vi "Obtain Request Events.vi"(8 "error in (no error)":errorcluster, 10 "Create New?":bool) -> (0 "error out":errorcluster, 2 "Anode Request Events":T1)   [LabVIEW 2024, in "Anode.lvlib"]
doc: "This VI Obtains/Creates the Requests events that will be used for other modules to communicate with the module that owns this VI. These Requests events will be accessed only via Public API methods for this module.\n\n<b>NOTE</b>: The contents of this VI are automatically generated and modified by the <b>Tools > Delacor > DQMH</b> utilities. Consider using those utilities instead of making your own modifications to this VI.\n_____\nBased on Delacor QMH Project Template 3.1.0.34."
uses:
  Anode.lvlib
  Request Events--cluster.ctl
  Stop Argument--cluster.ctl
  Show Panel Argument--cluster.ctl
  Hide Panel Argument--cluster.ctl
  Get Module Execution Status Argument--cluster.ctl
  Show Diagram Argument--cluster.ctl
  Change Panel Argument--cluster.ctl
  <vilib>/MGI/Panel Manager/Panel/Panel/Panel.lvclass
  Set Anode Inlet Pressure SP Argument--cluster.ctl
  Initialise Pressure Regulator Interface Argument--cluster.ctl
  Modbus Config--cluster.ctl
  Start Polling Pressure Regulator Status Argument--cluster.ctl
  Stop Polling Pressure Regulator Status Argument--cluster.ctl
  Read Pressure Regulator Status Argument--cluster.ctl
  Set Pressure Regulator Control Function Argument--cluster.ctl
  Modbus Flexi-Flow API/Control Function Values--enum.ctl
  Set Anode Inlet Flow SP Argument--cluster.ctl
  Set Anode Inlet Valve State Argument--cluster.ctl
  Anode Solenoid Valve--enum.ctl
  Wake Connection Helper Loop Argument--cluster.ctl
  Set Anode Gas Supply Valve Argument--cluster.ctl
  Set Purge Valve Argument--cluster.ctl
  Set Purge Strategy Argument--cluster.ctl
  Purge Strategy--cluster.ctl
  Purge Strategy--enum.ctl
  Wake Purge Strategy Helper Loop Argument--cluster.ctl
  Update Purge Strategy Settings Argument--cluster.ctl
  Wake Purge Helper Loop Argument--cluster.ctl
  Wake Recirculation Pump Helper Loop Argument--cluster.ctl
  Sleep Recirculation Pump Helper Loop Argument--cluster.ctl
  Set Pump Speed SP Argument--cluster.ctl
  Set Pump Enable State Argument--cluster.ctl
  Set Pump Speed Control Mode Argument--cluster.ctl
  Update Purge Strategy Helper Loop Argument--cluster.ctl
  Force Purge Argument--cluster.ctl
  Reset Counter Argument--cluster.ctl
  Wake H2 Sensor Loop Argument--cluster.ctl
  Sleep H2 Sensor Loop Argument--cluster.ctl
  Start H2 Sensor Measurement Argument--cluster.ctl
  Stop H2 Sensor Measurement Argument--cluster.ctl
  Modbus Flexi-Flow API/Bronkhorst Flexi-Flow ModbusTCP API.lvlib
panel:
  # "NOTE: The contents of this VI are automatically generated and modified by the Tools > Delacor > DQMH utilities. Consider using those utilities instead of making your own modifications to this VI."
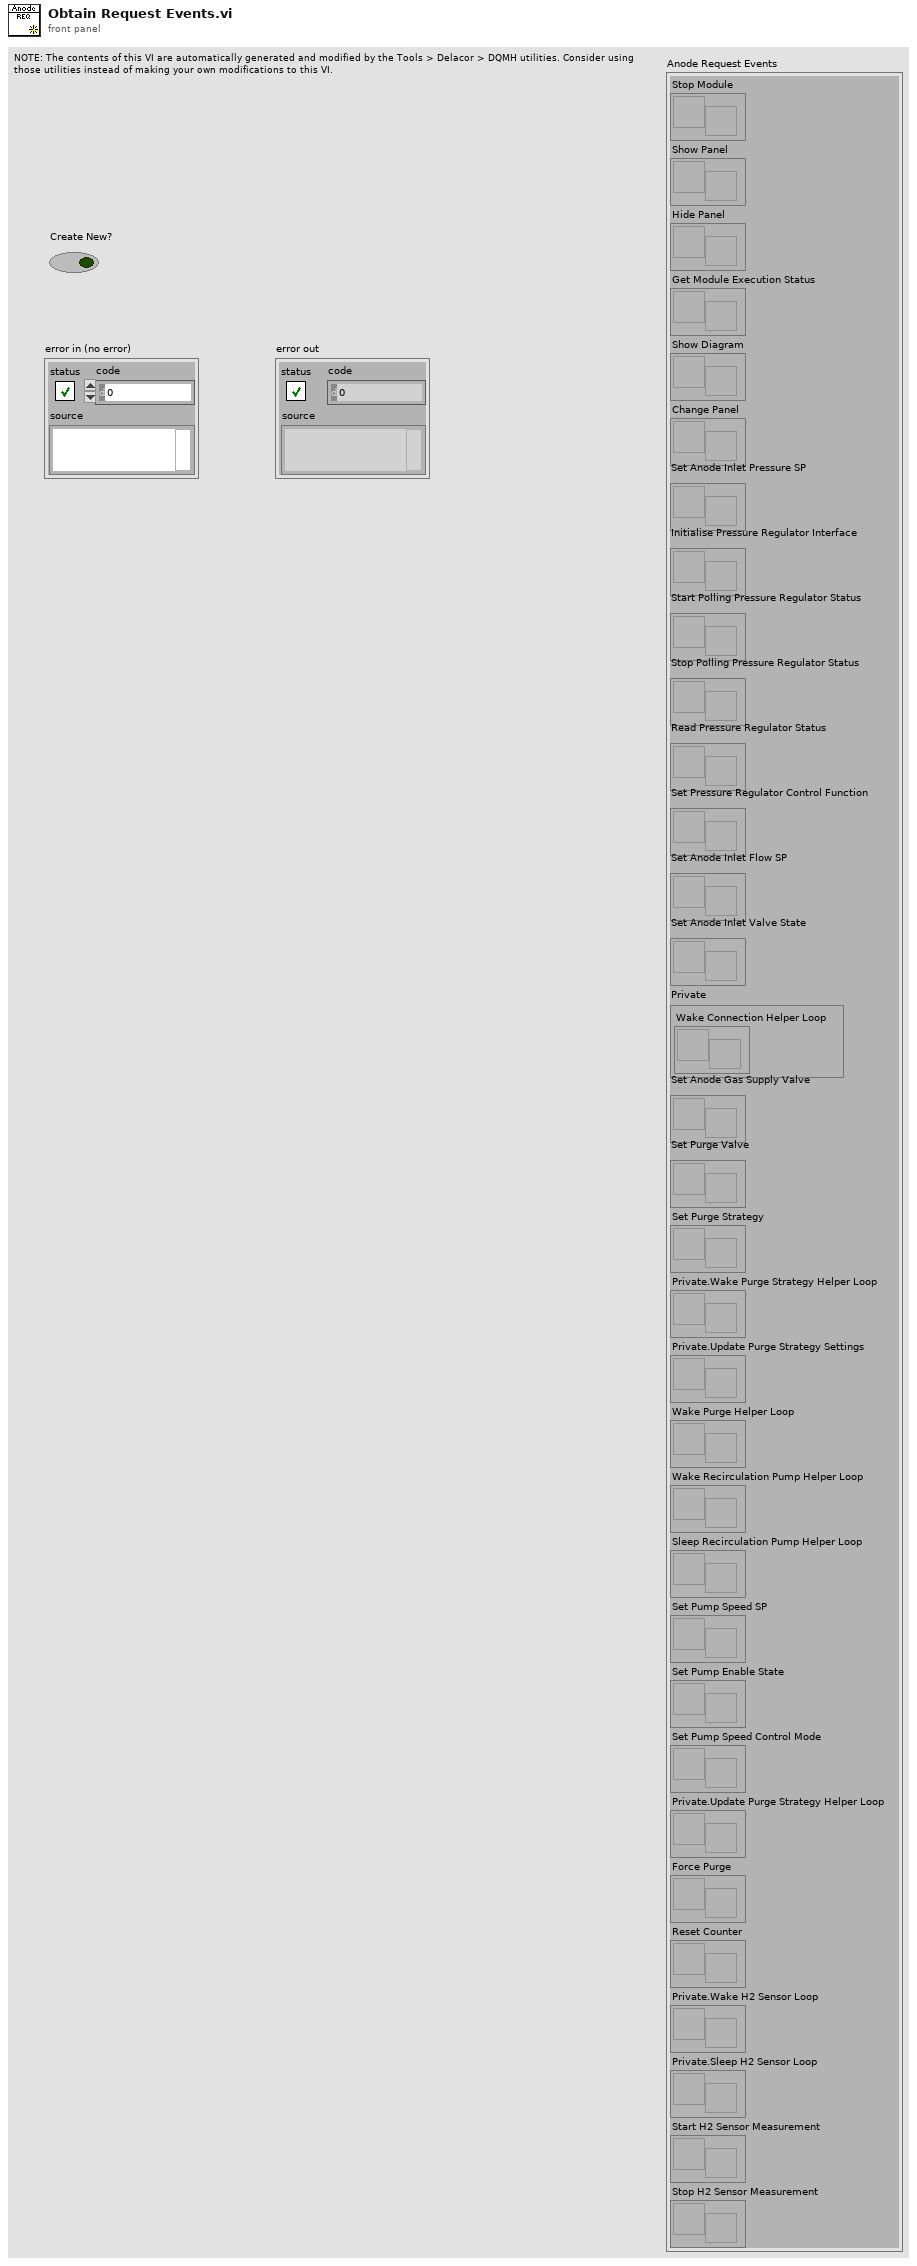
[diagram p1: front panel]
types:
  T1 = typedef "Anode.lvlib/Request Events--cluster.ctl" = cluster{"Stop Module":refnum<user-event>, "Show Panel":refnum<user-event>, "Hide Panel":refnum<user-event>, "Get Module Execution Status":refnum<user-event>, "Show Diagram":refnum<user-event>, "Change Panel":refnum<user-event>, "Set Anode Inlet Pressure SP":refnum<user-event>, "Initialise Pressure Regulator Interface":refnum<user-event>, "Start Polling Pressure Regulator Status":refnum<user-event>, "Stop Polling Pressure Regulator Status":refnum<user-event>, "Read Pressure Regulator Status":refnum<user-event>, "Set Pressure Regulator Control Function":refnum<user-event>, "Set Anode Inlet Flow SP":refnum<user-event>, "Set Anode Inlet Valve State":refnum<user-event>, "Private":cluster{"Wake Connection Helper Loop":refnum<user-event>}, "Set Anode Gas Supply Valve":refnum<user-event>, "Set Purge Valve":refnum<user-event>, "Set Purge Strategy":refnum<user-event>, "Private.Wake Purge Strategy Helper Loop":refnum<user-event>, "Private.Update Purge Strategy Settings":refnum<user-event>, "Wake Purge Helper Loop":refnum<user-event>, "Wake Recirculation Pump Helper Loop":refnum<user-event>, "Sleep Recirculation Pump Helper Loop":refnum<user-event>, "Set Pump Speed SP":refnum<user-event>, "Set Pump Enable State":refnum<user-event>, "Set Pump Speed Control Mode":refnum<user-event>, "Private.Update Purge Strategy Helper Loop":refnum<user-event>, "Force Purge":refnum<user-event>, "Reset Counter":refnum<user-event>, "Private.Wake H2 Sensor Loop":refnum<user-event>, "Private.Sleep H2 Sensor Loop":refnum<user-event>, "Start H2 Sensor Measurement":refnum<user-event>, "Stop H2 Sensor Measurement":refnum<user-event>}
  T2 = typedef "Anode.lvlib/Stop H2 Sensor Measurement Argument--cluster.ctl" = cluster{"Boolean":bool}
  T3 = typedef "Anode.lvlib/Start H2 Sensor Measurement Argument--cluster.ctl" = cluster{"Boolean":bool}
  T4 = typedef "Anode.lvlib/Sleep H2 Sensor Loop Argument--cluster.ctl" = cluster{"Boolean":bool}
  T5 = typedef "Anode.lvlib/Wake H2 Sensor Loop Argument--cluster.ctl" = cluster{"Boolean":bool}
  T6 = typedef "Anode.lvlib/Reset Counter Argument--cluster.ctl" = cluster{"Boolean":bool}
  T7 = typedef "Anode.lvlib/Force Purge Argument--cluster.ctl" = cluster{"Boolean":bool}
  T8 = typedef "Anode.lvlib/Update Purge Strategy Helper Loop Argument--cluster.ctl" = cluster{"Purge Controller":T9}
  T9 = typedef "Anode.lvlib/Purge Strategy--cluster.ctl" = cluster{"Strategy":T10, "Purge Interval [s]":dbl, "Purge Duration [s]":dbl}
  T10 = typedef "Anode.lvlib/Purge Strategy--enum.ctl" = enum16{"FORCE OFF", "FORCE ON", "TIMED"}
  T11 = typedef "Anode.lvlib/Set Pump Speed Control Mode Argument--cluster.ctl" = cluster{"Enable Speed Control":enum8{"DISABLE", "ENABLE"}}
  T12 = typedef "Anode.lvlib/Set Pump Enable State Argument--cluster.ctl" = cluster{"Enable Pump":enum16{"DISABLE", "ENABLE"}}
  T13 = typedef "Anode.lvlib/Set Pump Speed SP Argument--cluster.ctl" = cluster{"Pump Speed SP":dbl}
  T14 = typedef "Anode.lvlib/Sleep Recirculation Pump Helper Loop Argument--cluster.ctl" = cluster{"Boolean":bool}
  T15 = typedef "Anode.lvlib/Wake Recirculation Pump Helper Loop Argument--cluster.ctl" = cluster{"Boolean":bool}
  T16 = typedef "Anode.lvlib/Wake Purge Helper Loop Argument--cluster.ctl" = cluster{"Boolean":bool}
  T17 = typedef "Anode.lvlib/Update Purge Strategy Settings Argument--cluster.ctl" = cluster{"Purge Settings":T9}
  T18 = typedef "Anode.lvlib/Wake Purge Strategy Helper Loop Argument--cluster.ctl" = cluster{"Boolean":bool}
  T19 = typedef "Anode.lvlib/Set Purge Strategy Argument--cluster.ctl" = cluster{"Purge Controller":T9}
  T20 = typedef "Anode.lvlib/Set Purge Valve Argument--cluster.ctl" = cluster{"Valve State":enum16{"CLOSED", "OPEN"}}
  T21 = typedef "Anode.lvlib/Set Anode Gas Supply Valve Argument--cluster.ctl" = cluster{"Valve State":enum16{"CLOSED", "OPEN"}}
  T22 = typedef "Anode.lvlib/Wake Connection Helper Loop Argument--cluster.ctl" = cluster{"Boolean":bool}
  T23 = typedef "Anode.lvlib/Set Anode Inlet Valve State Argument--cluster.ctl" = cluster{"Anode Solenoid Valve":T24}
  T24 = typedef "Anode.lvlib/Anode Solenoid Valve--enum.ctl" = enum16{"CLOSED", "OPEN"}
  T25 = typedef "Anode.lvlib/Set Anode Inlet Flow SP Argument--cluster.ctl" = cluster{"Flow SP [slm]":dbl}
  T26 = typedef "Anode.lvlib/Set Pressure Regulator Control Function Argument--cluster.ctl" = cluster{"Function":T27}
  T27 = typedef "Bronkhorst Flexi-Flow ModbusTCP API.lvlib/Control Function Values--enum.ctl" = enum16{"Flow", "Upstream pressure", "Downstream pressure", "Flow with upstream pressure limit", "Flow with downstream pressure limit", "Upstream pressure with flow limit", "Downstream pressure with flow limit"}
  T28 = typedef "Anode.lvlib/Read Pressure Regulator Status Argument--cluster.ctl" = cluster{"Boolean":bool}
  T29 = typedef "Anode.lvlib/Stop Polling Pressure Regulator Status Argument--cluster.ctl" = cluster{"Boolean":bool}
  T30 = typedef "Anode.lvlib/Start Polling Pressure Regulator Status Argument--cluster.ctl" = cluster{"Polling Interval [ms]":i32}
  T31 = typedef "Anode.lvlib/Initialise Pressure Regulator Interface Argument--cluster.ctl" = cluster{"Modbus Config":T32}
  T32 = typedef "Anode.lvlib/Modbus Config--cluster.ctl" = cluster{"IP Address":string, "Port (502)":u16, "Slave ID (255)":u8, "Timeout (10000)":i32}
  T33 = typedef "Anode.lvlib/Set Anode Inlet Pressure SP Argument--cluster.ctl" = cluster{"Anode Inlet Pressure [bar]":dbl}
  T34 = typedef "Anode.lvlib/Change Panel Argument--cluster.ctl" = cluster{"New Panel":refnum<class "Panel.lvclass">}
  T35 = typedef "Anode.lvlib/Hide Panel Argument--cluster.ctl" = cluster{"Hide Panel?":bool}
  T36 = typedef "Anode.lvlib/Show Panel Argument--cluster.ctl" = cluster{"Show Panel?":bool}
  T37 = typedef "Anode.lvlib/Show Diagram Argument--cluster.ctl" = cluster{"Debug?":bool}
  T38 = typedef "Anode.lvlib/Get Module Execution Status Argument--cluster.ctl" = cluster{"Running?":bool}
  T39 = typedef "Anode.lvlib/Stop Argument--cluster.ctl" = cluster{"Origin":string, "Exit via Stop Module Req?":bool, "Wait for Module to stop?":bool}
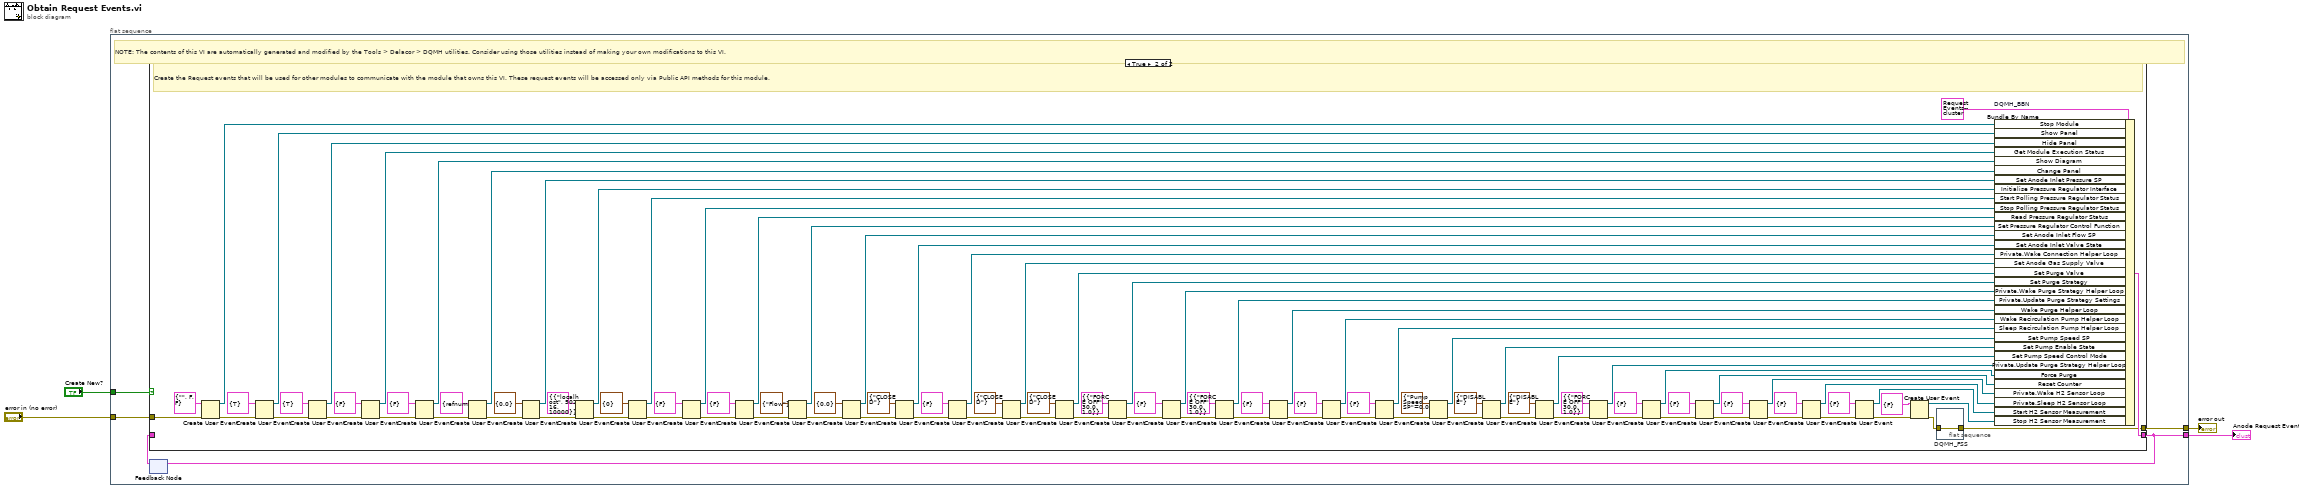
[diagram p0: block diagram]
diagram:
  n1 = flat-sequence {
    tunnel: [w9] -> w4
    tunnel: "error in (no error)" -> [w8]
    tunnel: [w6] -> w2
    tunnel: "Create New?" -> [w5]
    frame #0 {
      # "NOTE: The contents of this VI are automatically generated and modified by the Tools > Delacor > DQMH utilities. Consider using those utilities instead of making your own modifications to this VI."
      n2 = feedback #1() -> (w7:T1)  [unwired: 1 in]
      n3 = case shown="True" w5 {
        tunnel: [w10 w104] -> w9
        tunnel: w8 -> [w10 w114]
        tunnel: [w11 w111] -> w6
        tunnel: w7 -> [w11 _]
        frame False {
          # "Obtain the Request events that were created in a previous call to this VI."
        }
        frame True {
          # "Create the Request events that will be used for other modules to communicate with the module that owns this VI. These request events will be accessed only via Public API methods for this module."
          n4 = Create User Event(user event datatype=T39 {"Origin"="", "Exit via Stop Module Req?"=FALSE, "Wait for Module to stop?"=FALSE} ("Stop Argument"), error in=w114) -> (user event=w112:refnum<user-event>, error out=w109:errorcluster)
          n5 = Create User Event(user event datatype=T36 {"Show Panel?"=TRUE} ("Show Panel Argument"), error in=w109) -> (user event=w108:refnum<user-event>, error out=w107:errorcluster)
          n6 = Create User Event(user event datatype=T35 {"Hide Panel?"=TRUE} ("Hide Panel Argument"), error in=w107) -> (user event=w106:refnum<user-event>, error out=w105:errorcluster)
          n7 = Create User Event(user event datatype=T38 {"Running?"=FALSE} ("Get Module Execution Status Argument"), error in=w105) -> (user event=w102:refnum<user-event>, error out=w103:errorcluster)
          n8 = Create User Event(user event datatype=T37 {"Debug?"=FALSE} ("Show Diagram Argument"), error in=w103) -> (user event=w99:refnum<user-event>, error out=w100:errorcluster)
          n9 = Create User Event(user event datatype=T34 {"New Panel"=refnum} ("Change Panel Argument"), error in=w100) -> (user event=w94:refnum<user-event>, error out=w95:errorcluster)
          n10 = Create User Event(user event datatype=T33 {"Anode Inlet Pressure [bar]"=0.0} ("Set Anode Inlet Pressure SP Argument"), error in=w95) -> (user event=w91:refnum<user-event>, error out=w92:errorcluster)
          n11 = Create User Event(user event datatype=T31 {"Modbus Config"={"IP Address"="localhost", "Port (502)"=502, "Slave ID (255)"=16, "Timeout (10000)"=10000}} ("Initialise Pressure Regulator Interface Argument"), error in=w92) -> (user event=w88:refnum<user-event>, error out=w89:errorcluster)
          n12 = Create User Event(user event datatype=T30 {"Polling Interval [ms]"=0} ("Read Pressure Regulator Status Argument"), error in=w89) -> (user event=w85:refnum<user-event>, error out=w86:errorcluster)
          n13 = Create User Event(user event datatype=T29 {"Boolean"=FALSE} ("Stop Polling Pressure Regulator Status Argument"), error in=w86) -> (user event=w82:refnum<user-event>, error out=w83:errorcluster)
          n14 = Create User Event(user event datatype=T28 {"Boolean"=FALSE} ("Read Pressure Regulator Status Argument"), error in=w83) -> (user event=w79:refnum<user-event>, error out=w80:errorcluster)
          n15 = Create User Event(user event datatype=T26 {"Function"=enum."Flow"} ("Set Pressure Regulator Control Function Argument"), error in=w80) -> (user event=w76:refnum<user-event>, error out=w77:errorcluster)
          n16 = Create User Event(user event datatype=T25 {"Flow SP [slm]"=0.0} ("Set Anode Inlet Flow SP Argument"), error in=w77) -> (user event=w73:refnum<user-event>, error out=w74:errorcluster)
          n17 = Create User Event(user event datatype=T23 {"Anode Solenoid Valve"=enum."CLOSED"} ("Set Anode Inlet Solenoid Valve State Argument"), error in=w74) -> (user event=w70:refnum<user-event>, error out=w71:errorcluster)
          n18 = Create User Event(user event datatype=T22 {"Boolean"=FALSE} ("Wake Connection Helper Loop Argument"), error in=w71) -> (user event=w67:refnum<user-event>, error out=w68:errorcluster)
          n19 = Create User Event(user event datatype=T21 {"Valve State"=enum."CLOSED"} ("Set Anode Gas Supply Valve Argument"), error in=w68) -> (user event=w64:refnum<user-event>, error out=w65:errorcluster)
          n20 = Create User Event(user event datatype=T20 {"Valve State"=enum."CLOSED"} ("Set Purge Valve Argument"), error in=w65) -> (user event=w61:refnum<user-event>, error out=w62:errorcluster)
          n21 = Create User Event(user event datatype=T19 {"Purge Controller"={"Strategy"=enum."FORCE OFF", "Purge Interval [s]"=30.0, "Purge Duration [s]"=1.0}} ("Set Purge Strategy Argument"), error in=w62) -> (user event=w58:refnum<user-event>, error out=w59:errorcluster)
          n22 = Create User Event(user event datatype=T18 {"Boolean"=FALSE} ("Wake Purge Strategy Helper Loop Argument"), error in=w59) -> (user event=w55:refnum<user-event>, error out=w56:errorcluster)
          n23 = Create User Event(user event datatype=T17 {"Purge Settings"={"Strategy"=enum."FORCE OFF", "Purge Interval [s]"=30.0, "Purge Duration [s]"=1.0}} ("Update Purge Strategy Settings Argument"), error in=w56) -> (user event=w52:refnum<user-event>, error out=w53:errorcluster)
          n24 = Create User Event(user event datatype=T16 {"Boolean"=FALSE} ("Wake Purge Helper Loop Argument"), error in=w53) -> (user event=w49:refnum<user-event>, error out=w50:errorcluster)
          n25 = Create User Event(user event datatype=T15 {"Boolean"=FALSE} ("Wake Recirculation Pump Helper Loop Argument"), error in=w50) -> (user event=w46:refnum<user-event>, error out=w47:errorcluster)
          n26 = Create User Event(user event datatype=T14 {"Boolean"=FALSE} ("Sleep Recirculation Pump Helper Loop Argument"), error in=w47) -> (user event=w43:refnum<user-event>, error out=w44:errorcluster)
          n27 = Create User Event(user event datatype=T13 {"Pump Speed SP"=0.0} ("Set Pump Speed SP Argument"), error in=w44) -> (user event=w40:refnum<user-event>, error out=w41:errorcluster)
          n28 = Create User Event(user event datatype=T12 {"Enable Pump"=enum."DISABLE"} ("Set Pump Enable State Argument"), error in=w41) -> (user event=w37:refnum<user-event>, error out=w38:errorcluster)
          n29 = Create User Event(user event datatype=T11 {"Enable Speed Control"=enum."DISABLE"} ("Enable Pump Speed Control Argument"), error in=w38) -> (user event=w34:refnum<user-event>, error out=w35:errorcluster)
          n30 = Create User Event(user event datatype=T8 {"Purge Controller"={"Strategy"=enum."FORCE OFF", "Purge Interval [s]"=30.0, "Purge Duration [s]"=1.0}} ("Update Purge Strategy Helper Loop Argument"), error in=w35) -> (user event=w31:refnum<user-event>, error out=w32:errorcluster)
          n31 = Create User Event(user event datatype=T7 {"Boolean"=FALSE} ("Force Purge Argument"), error in=w32) -> (user event=w28:refnum<user-event>, error out=w29:errorcluster)
          n32 = Create User Event(user event datatype=T6 {"Boolean"=FALSE} ("Reset Counter Argument"), error in=w29) -> (user event=w25:refnum<user-event>, error out=w26:errorcluster)
          n33 = Create User Event(user event datatype=T5 {"Boolean"=FALSE} ("Wake H2 Sensor Loop Argument"), error in=w26) -> (user event=w22:refnum<user-event>, error out=w23:errorcluster)
          n34 = Create User Event(user event datatype=T4 {"Boolean"=FALSE} ("Sleep H2 Sensor Loop Argument"), error in=w23) -> (user event=w19:refnum<user-event>, error out=w20:errorcluster)
          n35 = Create User Event(user event datatype=T3 {"Boolean"=FALSE} ("Start H2 Sensor Measurement Argument"), error in=w20) -> (user event=w16:refnum<user-event>, error out=w17:errorcluster)
          n36 = Create User Event(user event datatype=T2 {"Boolean"=FALSE} ("Stop H2 Sensor Measurement Argument"), error in=w17) -> (user event=w13:refnum<user-event>, error out=w14:errorcluster)
          n37 = flat-sequence "DQMH_FSS" {
            tunnel: w14 -> [w115]
            tunnel: [w115] -> w104
            frame #0 {
            }
          }
          n38 = Bundle By Name "DQMH_BBN"(cluster=T1 {"Stop Module"=refnum, "Show Panel"=refnum, "Hide Panel"=refnum, "Get Module Execution Status"=refnum, "Show Diagram"=refnum, "Change Panel"=refnum, "Set Anode Inlet Pressure SP"=refnum, "Initialise Pressure Regulator Interface"=refnum, "Start Polling Pressure Regulator Status"=refnum, "Stop Polling Pressure Regulator Status"=refnum, "Read Pressure Regulator Status"=refnum, "Set Pressure Regulator Control Function"=refnum, "Set Anode Inlet Flow SP"=refnum, "Set Anode Inlet Valve State"=refnum, "Private"={"Wake Connection Helper Loop"=refnum}, "Set Anode Gas Supply Valve"=refnum, "Set Purge Valve"=refnum, "Set Purge Strategy"=refnum, "Private.Wake Purge Strategy Helper Loop"=refnum, "Private.Update Purge Strategy Settings"=refnum, "Wake Purge Helper Loop"=refnum, "Wake Recirculation Pump Helper Loop"=refnum, "Sleep Recirculation Pump Helper Loop"=refnum, "Set Pump Speed SP"=refnum, "Set Pump Enable State"=refnum, "Set Pump Speed Control Mode"=refnum, "Private.Update Purge Strategy Helper Loop"=refnum, "Force Purge"=refnum, "Reset Counter"=refnum, "Private.Wake H2 Sensor Loop"=refnum, "Private.Sleep H2 Sensor Loop"=refnum, "Start H2 Sensor Measurement"=refnum, "Stop H2 Sensor Measurement"=refnum} ("output cluster"), "Stop Module"=w112, "Show Panel"=w108, "Hide Panel"=w106, "Get Module Execution Status"=w102, "Show Diagram"=w99, "Change Panel"=w94, "Set Anode Inlet Pressure SP"=w91, "Initialise Pressure Regulator Interface"=w88, "Start Polling Pressure Regulator Status"=w85, "Stop Polling Pressure Regulator Status"=w82, "Read Pressure Regulator Status"=w79, "Set Pressure Regulator Control Function"=w76, "Set Anode Inlet Flow SP"=w73, "Set Anode Inlet Valve State"=w70, "Private.Wake Connection Helper Loop"=w67, "Set Anode Gas Supply Valve"=w64, "Set Purge Valve"=w61, "Set Purge Strategy"=w58, "Private.Wake Purge Strategy Helper Loop"=w55, "Private.Update Purge Strategy Settings"=w52, "Wake Purge Helper Loop"=w49, "Wake Recirculation Pump Helper Loop"=w46, "Sleep Recirculation Pump Helper Loop"=w43, "Set Pump Speed SP"=w40, "Set Pump Enable State"=w37, "Set Pump Speed Control Mode"=w34, "Private.Update Purge Strategy Helper Loop"=w31, "Force Purge"=w28, "Reset Counter"=w25, "Private.Wake H2 Sensor Loop"=w22, "Private.Sleep H2 Sensor Loop"=w19, "Start H2 Sensor Measurement"=w16, "Stop H2 Sensor Measurement"=w13) -> (w111:T1)
        }
      }
      n39 = feedback-in #1(w6) -> ()
    }
  }
  "Anode Request Events" <- w2
  "error out" <- w4
